vi "Bool_Edge Detect.vi"(9 "Initial State":bool, 11 "Input/Set":bool) -> (0 "Change":bool, 1 "Fall":bool, 2 "Rise":bool, 3 "Output":bool)   [LabVIEW 2020]
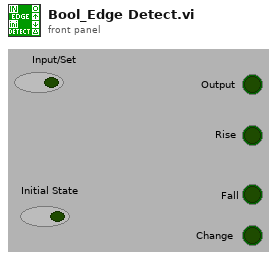
[diagram p1: front panel]
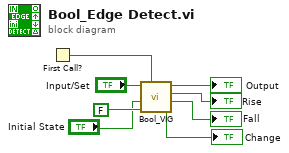
[diagram p0: block diagram]
diagram:
  n1 = First Call?() -> (First Call?: T/F=w2:bool)
  n2 = call "Bool_VIG.vi"("First call"=w2, "Latch(t) Edge(f)"=FALSE, "Initial State"="Initial State", "Input/Set"="Input/Set") -> ("Change"=→"Change":bool, "Fall"=→"Fall":bool, "Rise"=→"Rise":bool, "Output"=→"Output":bool)  [unwired: 4 in]
